vi "FileEnumerator.vi"(4 "Filename":string, 5 "Path":path) -> (0 "Number":i32, 1 "Filename+Number":string, 2 "appended path":path)   [LabVIEW 2009]
doc: "Useful program to create new files.\nChecks for a file name under a certain path. If the filename exists it either appends a number to it , or increments the number (if one already exists). Keeps the file extension in tact. Returns both the path, the new string, and the number appended.\nGreat for sequential trials, etc."
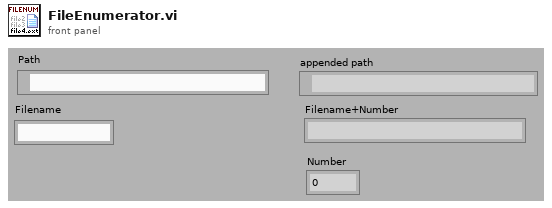
[diagram p1: front panel]
types:
  T1 = enum16{"open", "replace", "create", "open or create", "replace or create", "replace or create with confirmation"}
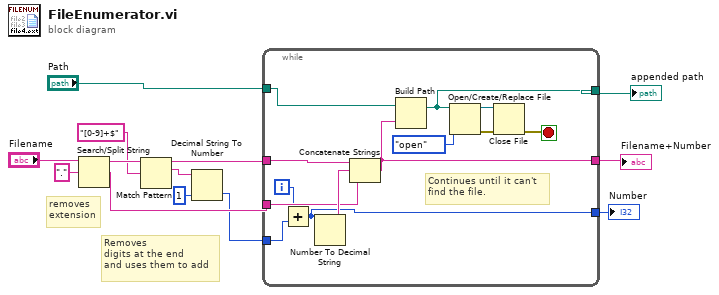
[diagram p0: block diagram]
diagram:
  # "Removes\ndigits at the end\nand uses them to add"
  # "removes\nextension"
  n1 = Search/Split String(string="Filename", search string/char (-)=".") -> (substring before match=w7:string, match + rest of string=w9:string)  [unwired: 1 in, 1 out]
  n2 = Match Pattern(string=w7, regular expression="[0-9]+$") -> (before substring=w6:string, match substring=w4:string)  [unwired: 1 in, 2 out]
  n3 = Decimal String To Number(string=w4, default (0L)=1 ("default (0 I32)")) -> (number=w2:i32)  [unwired: 1 in, 1 out]
  n4 = while {
    tunnel: w6 -> [w25]
    tunnel: "Path" -> [w24]
    tunnel: [w22] -> w12
    tunnel: [w21] -> w8
    tunnel: w9 -> [w20]
    tunnel: w2 -> [w16]
    tunnel: [w14] -> w1
    i -> [w15]
    stop <- w17 stop-if-true
    # "Continues until it can't\nfind the file."
    n5 = Add(x=w15, y=w16) -> (x+y=w14:i32)
    n6 = Number To Decimal String(number=w14) -> (decimal integer string=w26:string)  [unwired: 1 in]
    n7 = Concatenate Strings(w25, w26, w20) -> (w21:string)
    n8 = Build Path(base path=w24, name or relative path=w21) -> (appended path=w22:path)
    n9 = Open/Create/Replace File(file path (use dialog)=w22, operation (0:open)=T1."open") -> (refnum out=w19:refnum<file>, error out=w18:errorcluster)  [unwired: 4 in, 1 out]
    n10 = Close File(refnum=w19, error in=w18) -> (error out=w17:errorcluster)  [unwired: 1 out]
  }
  "appended path" <- w12
  "Filename+Number" <- w8
  "Number" <- w1
